vi "Set Report Footer Text.vi"(0 "report in":refnum<class "NI_HTML.lvclass">, 5 "left footer text":string, 7 "center footer text":string, 9 "right footer text":string, 11 "error in (no error)":errorcluster, 12 "HTML footer size":enum16{"H1", "H2", "H3", "H4", "H5", "H6", "H7"}(ring)=enum."H3") -> (4 "report out":refnum<class "NI_HTML.lvclass">, 15 "error out":errorcluster)   [LabVIEW 2017, in "NI_HTML.lvclass"]
doc: "Sets the text of the report footer."
uses:
  <vilib>/Utility/NIReport.llb/HTML/NI_HTML.lvclass
  <vilib>/Utility/NIReport.llb/HTML/NI_HTML.lvclass/NI_HTML.ctl
  <vilib>/Utility/NIReport.llb/NI_ReportGenerationCore.lvlib
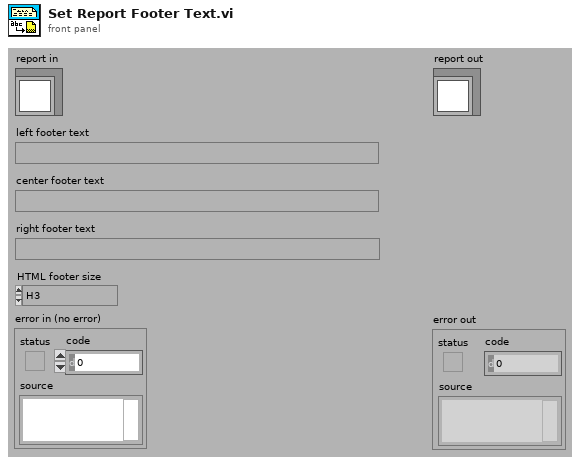
[diagram p1: front panel]
types:
  T1 = typedef "NI_ReportGenerationCore.lvlib/HTML Report Data.ctl" = cluster{"Body Text":string, "Font Tag":string, "Title Text":string, "Header Text":string, "Footer Text":string, "Image List":path[]}
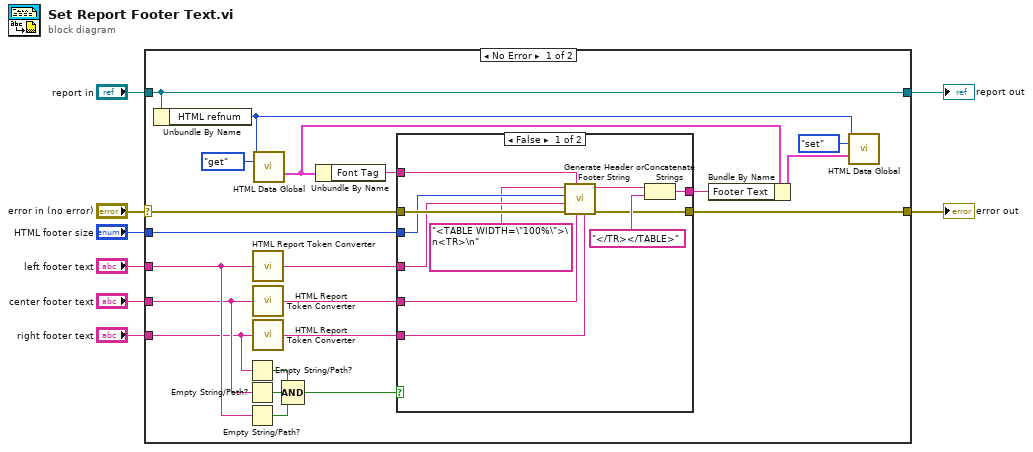
[diagram p0: block diagram]
diagram:
  n1 = case shown="No Error" "error in (no error)" {
    selector: "error in (no error)" -> [w16 w43]
    tunnel: [w15 w43] -> w7
    tunnel: [w13 w42] -> w5
    tunnel: "report in" -> [w13 w42]
    tunnel: "left footer text" -> [w20 _]
    tunnel: "center footer text" -> [w19 _]
    tunnel: "right footer text" -> [w18 _]
    tunnel: "HTML footer size" -> [w17 _]
    frame No Error {
      n2 = Unbundle By Name(w13) -> ("HTML refnum"=w9:u32)
      n3 = Empty String/Path?(string/path=w18) -> (empty?=w23:bool)
      n4 = Empty String/Path?(string/path=w19) -> (empty?=w24:bool)
      n5 = Empty String/Path?(string/path=w20) -> (empty?=w25:bool)
      n6 = call <vilib>:"HTML Report Token Converter.vi"("String In"=w20) -> ("String Out"=w26:string)
      n7 = call <vilib>:"HTML Report Token Converter.vi"("String In"=w19) -> ("String Out"=w29:string)
      n8 = call <vilib>:"HTML Report Token Converter.vi"("String In"=w18) -> ("String Out"=w27:string)
      n9 = call <vilib>:"HTML Data Global.vi"("HTML refnum"=w9, "menu"=enum16{"init", "get", "set", "delete"}."get") -> ("HTML report data out"=w12:T1)  [unwired: 1 in, 12 out]
      n10 = Compound Arithmetic op=AND(w23, w24, w25) -> (w28:bool)
      n11 = Unbundle By Name(w12) -> ("Font Tag"=w22:string)
      n12 = case shown="False" w28 {
        tunnel: w26 -> [w35 _]
        tunnel: w29 -> [w34 _]
        tunnel: w27 -> [w33 _]
        tunnel: [w32 w41] -> w15
        tunnel: w16 -> [w38 w41]
        tunnel: w22 -> [w37 _]
        tunnel: w17 -> [w36 _]
        tunnel: [w40 _] -> w21
        frame False {
          n13 = call <vilib>:"Generate Header or Footer String.vi"("Right Text"=w33, "Center Text"=w34, "Font Tag"=w37, "error in (no error)"=w38, "Left Text"=w35, "size"=w36, "HTML in"="<TABLE WIDTH=\"100%\">\n<TR>\n" ("Substring")) -> ("error out"=w32:errorcluster, "HTML out"=w30:string)  [unwired: 3 out]
          n14 = Concatenate Strings(w30, "</TR></TABLE>" ("Substring")) -> (w40:string)
        }
        frame True {
        }
      }
      n15 = Bundle By Name(cluster=w12, "Footer Text"=w21) -> (w10:T1)
      n16 = call <vilib>:"HTML Data Global.vi"("HTML refnum"=w9, "menu"=enum16{"init", "get", "set", "delete"}."set", "HTML report data in"=w10) -> ()  [unwired: 13 out]
    }
    frame Error {
    }
  }
  "error out" <- w7
  "report out" <- w5
